vi "Register.vi"() -> ()   [LabVIEW 2015]
uses:
  GlobalVar.vi
panel:
  in  "LicenseIn":string caption="License:"
  in  "btnSignup":bool
  in  "btnPasteLicense":bool
  in  "btnClose":bool
  in  "btnCopyUID":bool
  out "UID":string caption="UID:"
  in  "License":string caption="License:"
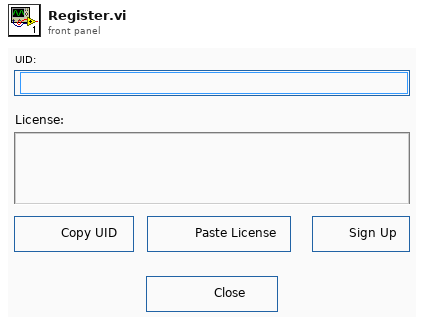
[diagram p1: front panel]
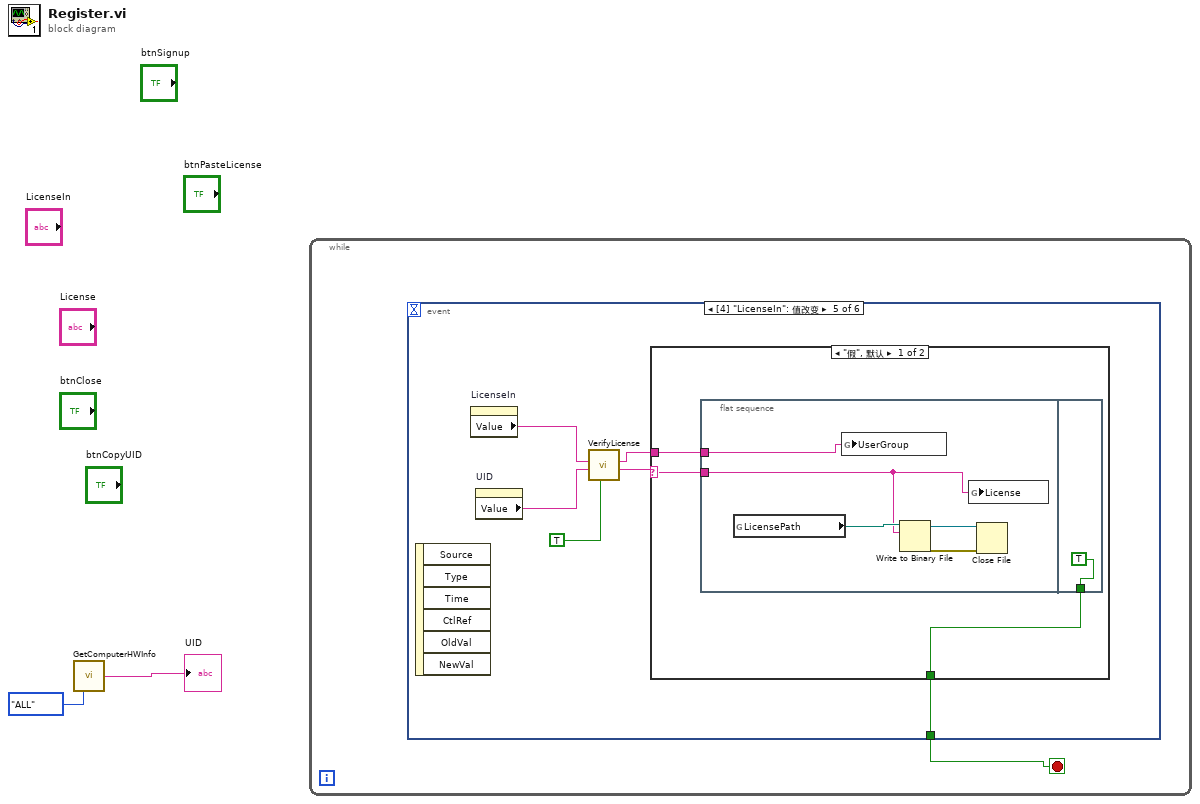
[diagram p0: block diagram]
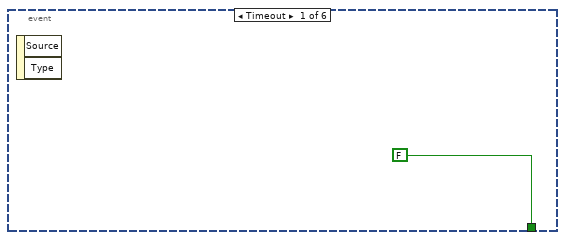
[diagram p2: hidden frame]
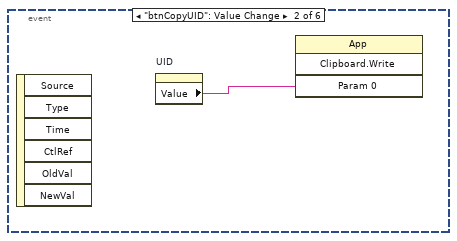
[diagram p3: hidden frame]
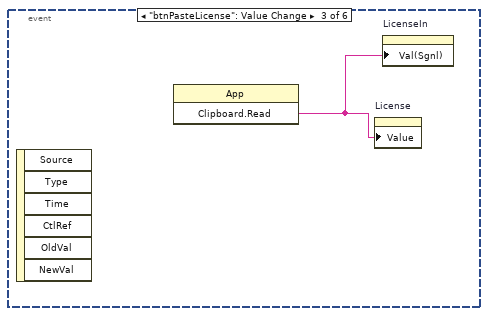
[diagram p4: hidden frame]
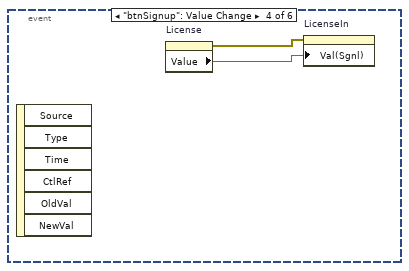
[diagram p5: hidden frame]
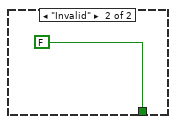
[diagram p6: hidden frame]
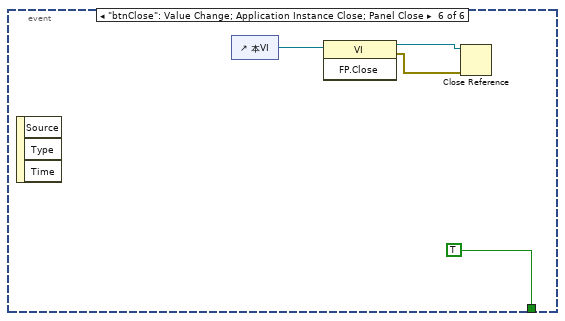
[diagram p7: hidden frame]
diagram:
  n1 = call "GetComputerHWInfo.vi"("获取内容"=enum16{"ALL", "HDD SN", "HDD Type", "MAC Adr"}."ALL") -> ("UID"=→"UID":string)  [unwired: 13 in, 1 out]
  n2 = while {
    stop <- w3 stop-if-true
    n3 = event shown="[4] \"LicenseIn\": 值改变" {
      selector: _ -> [_ _ _ _ _ _]
      dyn-events: _ -> [_ _ _ _ _ _]
      timeout: _ -> [_ _ _ _ _ _]
      tunnel: [FALSE _ _ _ w9 TRUE] -> w3
      event Timeout {
        n4 = event-data() -> ()  [unwired: 1 in, 2 out]
      }
      event "btnCopyUID": Value Change {
        n5 = event-data() -> ()  [unwired: 1 in, 6 out]
        n6 = property on="UID" class="Str"() -> ("Value"=w5:string)  [unwired: 2 in, 2 out]
        n7 = invoke class="App" method="Clipboard.Write"("Param 0"=w5) -> ()  [unwired: 3 in, 4 out]
      }
      event "btnPasteLicense": Value Change {
        n8 = event-data() -> ()  [unwired: 1 in, 6 out]
        n9 = invoke class="App" method="Clipboard.Read"() -> ("Read Clipbrd"=w6:string)  [unwired: 3 in, 2 out]
        n10 = property on="License" class="Str"("Value"=w6) -> ()  [unwired: 2 in, 2 out]
        n11 = property on="LicenseIn" class="Str"("Val(Sgnl)"=w6) -> ()  [unwired: 2 in, 2 out]
      }
      event "btnSignup": Value Change {
        n12 = event-data() -> ()  [unwired: 1 in, 6 out]
        n13 = property on="License" class="Str"() -> (error out=w7:errorcluster, "Value"=w8:string)  [unwired: 2 in, 1 out]
        n14 = property on="LicenseIn" class="Str"(error in=w7, "Val(Sgnl)"=w8) -> ()  [unwired: 1 in, 2 out]
      }
      event "LicenseIn": Value Change {
        n15 = event-data() -> ()  [unwired: 1 in, 6 out]
        n16 = property on="LicenseIn" class="Str"() -> ("Value"=w13:string)  [unwired: 2 in, 2 out]
        n17 = property on="UID" class="Str"() -> ("Value"=w14:string)  [unwired: 2 in, 2 out]
        n18 = call "VerifyLicense.vi"("Tips"=TRUE, "UID"=w14, "License"=w13) -> ("LicenOut"=w11:string, "user"=w10:string)  [unwired: 7 in]
        n19 = case shown="\"假\", 默认" w11 {
          selector: w11 -> [w16 _]
          tunnel: w10 -> [w17 _]
          tunnel: [w15 FALSE] -> w9
          frame "假", Default {
            n20 = flat-sequence {
              tunnel: w17 -> [w22]
              tunnel: w16 -> [w18]
              tunnel: [TRUE] -> w15
              frame #0 {
                n21 = global read "GlobalVar.vi" "LicensePath"() -> (w21:path)
                n22 = global write "GlobalVar.vi" "UserGroup"(w22) -> ()
                n23 = Write to Binary File(file (use dialog)=w21, data=w18) -> (refnum out=w20:refnum<file>, error out=w19:errorcluster)  [unwired: 4 in, 1 out]
                n24 = global write "GlobalVar.vi" "License"(w18) -> ()
                n25 = Close File(refnum=w20, error in=w19) -> ()  [unwired: 2 out]
              }
              frame #1 {
              }
            }
          }
          frame "Invalid" {
          }
        }
      }
      event "btnClose": Value Change; Application Instance Close; Panel Close {
        n26 = event-data() -> ()  [unwired: 1 in, 3 out]
        n27 = control-ref of="本VI"() -> (w28:refnum<vi>)
        n28 = invoke class="VI" method="FP.Close"(reference=w28) -> (reference out=w27:refnum<vi>, error out=w26:errorcluster)  [unwired: 2 in, 1 out]
        n29 = Close Reference(reference=w27, error in (no error)=w26) -> ()  [unwired: 1 out]
      }
    }
  }
